vi "VI Main 1.1GPIB.vi"() -> ()   [LabVIEW 2014]
uses:
  <vilib>/Analysis/NI_AALPro.lvlib
panel:
  in  "clear graph at start":bool=TRUE
  in  "clear graph":bool
  out "Elapsed Time":dbl=5.100291728973389 format="%<%H:%M:%S>t"
  out "Measuring!":bool
  out "Current Interval":i32=2
  out "Benchmark (s)":dbl=1.077 format="%.2g"
  out "Start time":timestamp=timestamp(3634319869.0891385 s since 1904-01-01)
  in  "STOP acq":bool
  in  "# of Intervals":i32=20 min=2 step=1
  in  "Interval (s)":dbl=3.0 min=1.0 step=1.0
  in  "Quick Acq":bool
  in  "Multi Acq":bool
  in  "Reset":bool
  in  "Single Acq":bool
  in  "stop":bool
  out "intercept":dbl=5.632151768673284e-07 format="%_4g"
  out "Waveform Chart":dbl(graph)=1498.8953969009954
  out "Res. (ohm)":dbl=1498.8953969009954 format="%#.5g"
  out "XY Graph":cluster{dbl[], "Best Linear Fit":dbl[]}[](graph)=[{[0.0, 0.05050000175833702, 0.10100000351667404, 0.15150000154972076, 0.20200000703334808, 0.2524999976158142, 0.30300000309944153, 0.35350000858306885, 0.40400001406669617, 0.4544999897480011, 0.5049999952316284, 0.5554999709129333, 0.6060000061988831, 0.656499981880188, 0.7070000171661377, 0.7574999928474426, 0.8080000281333923, 0.8585000038146973, 0.9089999794960022, 0.9595000147819519, 1.0099999904632568, 1.0605000257492065, 1.1109999418258667, 1.1614999771118164, 1.2120000123977661, 1.2625000476837158, 1.312999963760376, 1.3634999990463257, 1.4140000343322754, 1.4644999504089355, 1.5149999856948853, 1.565500020980835, 1.6160000562667847, 1.6664999723434448, 1.7170000076293945, 1.7675000429153442, 1.8179999589920044, 1.868499994277954, 1.9190000295639038, 1.969499945640564, 2.0199999809265137, 2.070499897003174, 2.121000051498413, 2.1714999675750732, 2.2219998836517334, 2.2725000381469727, 2.322999954223633, 2.373500108718872, 2.4240000247955322, 2.4744999408721924, 2.5255000591278076, 2.5759999752044678, 2.626499891281128, 2.677000045776367, 2.7274999618530273, 2.7780001163482666, 2.8285000324249268, 2.878999948501587, 2.929500102996826, 2.9800000190734863, 3.0304999351501465, 3.0810000896453857, 3.131500005722046, 3.181999921798706, 3.2325000762939453, 3.2829999923706055, 3.3334999084472656, 3.384000062942505, 3.434499979019165, 3.484999895095825, 3.5355000495910645, 3.5859999656677246, 3.6364998817443848, 3.687000036239624, 3.737499952316284, 3.7880001068115234, 3.8385000228881836, 3.8889999389648438, 3.939500093460083, 3.990000009536743, 4.040500164031982, 4.091000080108643, 4.141499996185303, 4.191999912261963, 4.242499828338623, 4.293000221252441, 4.343500137329102, 4.394000053405762, 4.444499969482422, 4.494999885559082, 4.545499801635742, 4.5960001945495605, 4.646500110626221, 4.697000026702881, 4.747499942779541, 4.797999858856201, 4.848499774932861, 4.89900016784668, 4.94950008392334, 5.0], "Best Linear Fit"=[2.9321361694201187e-07, 3.4316144592594355e-05, 6.788442260585725e-05, 0.00010163152910536155, 0.0001353666593786329, 0.0001692490477580577, 0.00020289691747166216, 0.0002365230757277459, 0.0002702110796235502, 0.0003039317671209574, 0.0003375497763045132, 0.00037135041202418506, 0.00040501810144633055, 0.000438651826698333, 0.0004723611054942012, 0.0005059913382865489, 0.0005397166823968291, 0.0005734616424888372, 0.0006071235402487218, 0.0006408520275726914, 0.000674474285915494, 0.0007079437491483986, 0.0007418016903102398, 0.0007753406534902751, 0.0008092316566035151, 0.0008428616565652192, 0.0008766247192397714, 0.0009101884788833559, 0.0009441068395972252, 0.000977773917838931, 0.0010113242315128446, 0.00104525254573673, 0.0010786742204800248, 0.0011119291884824634, 0.0011458882363513112, 0.0011792887235060334, 0.0012128128437325358, 0.001246674102731049, 0.0012809749459847808, 0.0013138956855982542, 0.0013484194641932845, 0.0013821402098983526, 0.001415521022863686, 0.0014488088199868798, 0.0014823464443907142, 0.0015171199338510633, 0.0015507071511819959, 0.0015843959990888834, 0.0016174258198589087, 0.001652282546274364, 0.001685628667473793, 0.001718429964967072, 0.0017526380252093077, 0.0017857326893135905, 0.0018194534350186586, 0.001854273141361773, 0.0018880483694374561, 0.0019207267323508859, 0.0019549881108105183, 0.001989204902201891, 0.0020224947948008776, 0.002056337194517255, 0.0020900650415569544, 0.0021233297884464264, 0.0021574627608060837, 0.0021917179692536592, 0.0022237151861190796, 0.002258580643683672, 0.0022912463173270226, 0.0023252873215824366, 0.0023596647661179304, 0.0023923530243337154, 0.0024269770365208387, 0.0024603772908449173, 0.002494191052392125, 0.0025280059780925512, 0.0025607654824852943, 0.0025952423457056284, 0.0026286595966666937, 0.0026625576429069042, 0.002696041017770767, 0.002730145351961255, 0.0027635691221803427, 0.0027978394646197557, 0.00283193145878613, 0.0028640953823924065, 0.002898684237152338, 0.0029313690029084682, 0.002965638181194663, 0.0029995907098054886, 0.0030326275154948235, 0.0030669174157083035, 0.003100987756624818, 0.003135110717266798, 0.0031680287793278694, 0.0032008818816393614, 0.0032355813309550285, 0.003269442357122898, 0.0033022440038621426, 0.0033363213296979666]}, {[0.0, 0.05050000175833702, 0.10100000351667404, 0.15150000154972076, 0.20200000703334808, 0.2524999976158142, 0.30300000309944153, 0.35350000858306885, 0.40400001406669617, 0.4544999897480011, 0.5049999952316284, 0.5554999709129333, 0.6060000061988831, 0.656499981880188, 0.7070000171661377, 0.7574999928474426, 0.8080000281333923, 0.8585000038146973, 0.9089999794960022, 0.9595000147819519, 1.0099999904632568, 1.0605000257492065, 1.1109999418258667, 1.1614999771118164, 1.2120000123977661, 1.2625000476837158, 1.312999963760376, 1.3634999990463257, 1.4140000343322754, 1.4644999504089355, 1.5149999856948853, 1.565500020980835, 1.6160000562667847, 1.6664999723434448, 1.7170000076293945, 1.7675000429153442, 1.8179999589920044, 1.868499994277954, 1.9190000295639038, 1.969499945640564, 2.0199999809265137, 2.070499897003174, 2.121000051498413, 2.1714999675750732, 2.2219998836517334, 2.2725000381469727, 2.322999954223633, 2.373500108718872, 2.4240000247955322, 2.4744999408721924, 2.5255000591278076, 2.5759999752044678, 2.626499891281128, 2.677000045776367, 2.7274999618530273, 2.7780001163482666, 2.8285000324249268, 2.878999948501587, 2.929500102996826, 2.9800000190734863, 3.0304999351501465, 3.0810000896453857, 3.131500005722046, 3.181999921798706, 3.2325000762939453, 3.2829999923706055, 3.3334999084472656, 3.384000062942505, 3.434499979019165, 3.484999895095825, 3.5355000495910645, 3.5859999656677246, 3.6364998817443848, 3.687000036239624, 3.737499952316284, 3.7880001068115234, 3.8385000228881836, 3.8889999389648438, 3.939500093460083, 3.990000009536743, 4.040500164031982, 4.091000080108643, 4.141499996185303, 4.191999912261963, 4.242499828338623, 4.293000221252441, 4.343500137329102, 4.394000053405762, 4.444499969482422, 4.494999885559082, 4.545499801635742, 4.5960001945495605, 4.646500110626221, 4.697000026702881, 4.747499942779541, 4.797999858856201, 4.848499774932861, 4.89900016784668, 4.94950008392334, 5.0], "Best Linear Fit"=[5.632151768673284e-07, 3.425469348999516e-05, 6.794617180312299e-05, 0.00010163764763089373, 0.00013532912842937865, 0.0001690205992864352, 0.00020271208008492013, 0.00023640356088340506, 0.00027009504168188996, 0.0003037865025975182, 0.0003374779833960031, 0.00037116944431163135, 0.0004048609449929729, 0.00043855240590860115, 0.0004722439065899428, 0.000505935367505571, 0.0005396268681869126, 0.0005733183291025409, 0.0006070097900181691, 0.0006407012906995107, 0.0006743927516151388, 0.0007080842522964805, 0.0007417756734463953, 0.0007754671741277369, 0.0008091586748090786, 0.0008428501754904202, 0.000876541596640335, 0.0009102330973216766, 0.0009439245980030183, 0.000977616019152933, 0.0010113075198342747, 0.0010449990205156163, 0.001078690521196958, 0.0011123819423468728, 0.0011460734430282144, 0.001179764943709556, 0.0012134563648594707, 0.0012471478655408123, 0.001280839366222154, 0.0013145307873720688, 0.0013482222880534104, 0.0013819137092033252, 0.0014156052894160936, 0.0014492967105660085, 0.0014829881317159233, 0.0015166797119286917, 0.0015503711330786066, 0.001584062713291375, 0.0016177541344412898, 0.0016514455555912046, 0.0016854706906080038, 0.0017191621117579187, 0.0017528535329078335, 0.001786545113120602, 0.0018202365342705167, 0.0018539281144832852, 0.0018876195356332, 0.0019213109567831148, 0.001955002536995883, 0.001988693958145798, 0.0020223853792957127, 0.0020560769595084813, 0.002089768380658396, 0.002123459801808311, 0.002157151382021079, 0.0021908428031709943, 0.002224534224320909, 0.0022582258045336775, 0.002291917225683592, 0.002325608646833507, 0.0023593002270462754, 0.00239299164819619, 0.002426683069346105, 0.0024603746495588733, 0.0024940660707087883, 0.0025277576509215565, 0.0025614490720714716, 0.002595140493221386, 0.002628832073434155, 0.0026625234945840694, 0.002696215074796838, 0.0027299064959467527, 0.0027635979170966677, 0.0027972893382465823, 0.0028309807593964974, 0.002864672498672119, 0.0028983639198220342, 0.002932055340971949, 0.002965746762121864, 0.0029994381832717785, 0.0030331296044216935, 0.0030668213436973154, 0.0031005127648472304, 0.003134204185997145, 0.0031678956071470596, 0.0032015870282969747, 0.0032352784494468893, 0.0032689701887225115, 0.003302661609872426, 0.003336353031022341]}]
  in  "Sense range":i32(slide)
  in  "Stop (V)":dbl=5.0 format="%.4f"
  in  "Source compliance (A)":dbl=0.01 format="%.4f"
  in  "Direction":i32(slide)
  in  "Ranging":i32(slide)
  in  "Start (V)":dbl step=1.0 format="%.4p"
  in  "# of points to acquire":i32=50 min=1 max=2500 step=1
  in  "Speed":i32(slide)=2
  out "status":i32 format="%.0x"
  in  "resource name 2":string="GPIB0::24::INSTR"
  in  "resource name":string="ASRL4::INSTR"
  out "Qrun":bool
  out "Mrun":bool
  out "Srun":bool
  # ">"
  # "by L.Andrzejewski\nlandrzej@uottawa.ca"
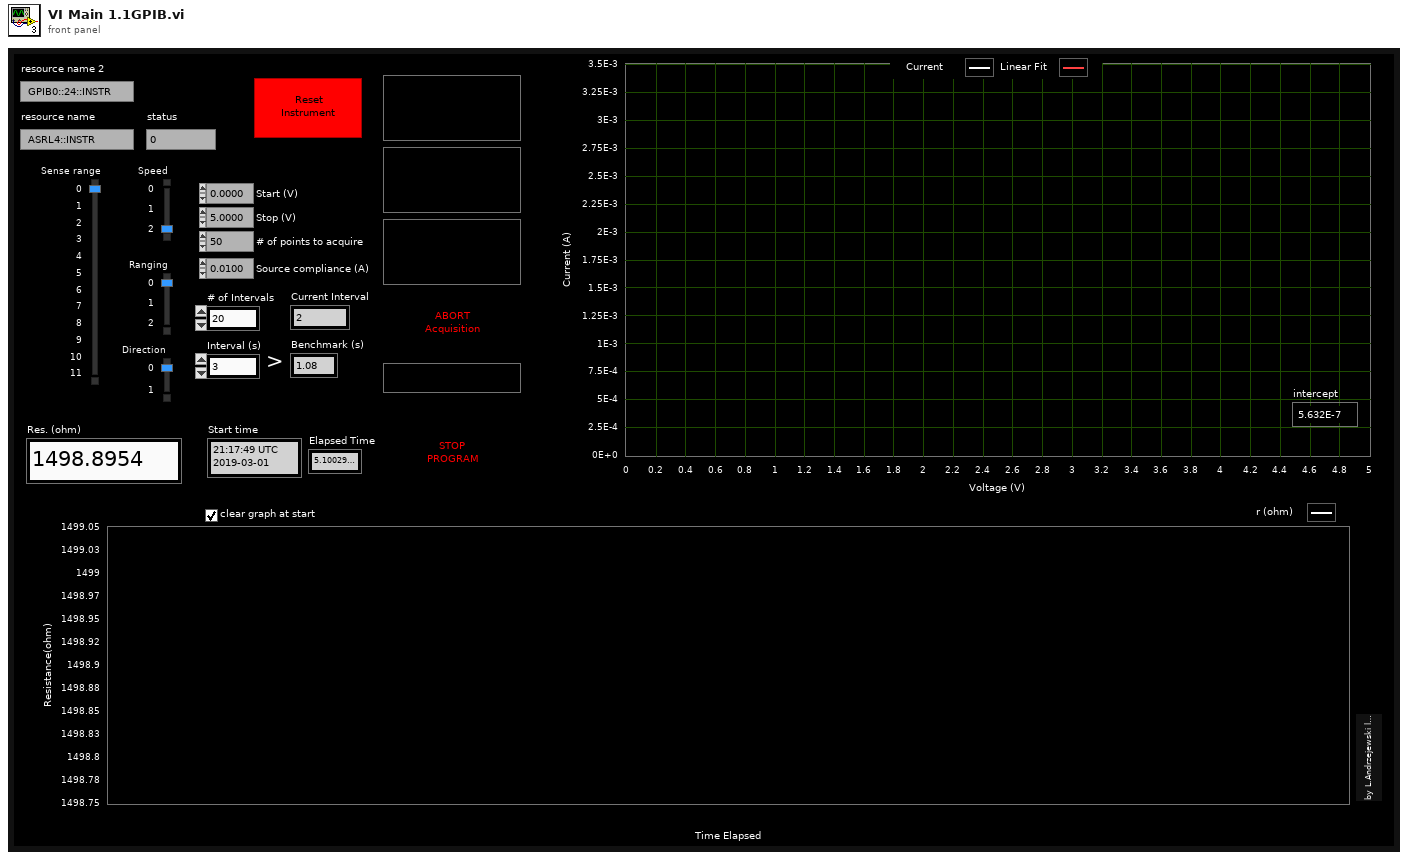
[diagram p1: front panel]
types:
  T1 = enum8{"Enabled", "Disabled", "Disabled and Grayed Out"}
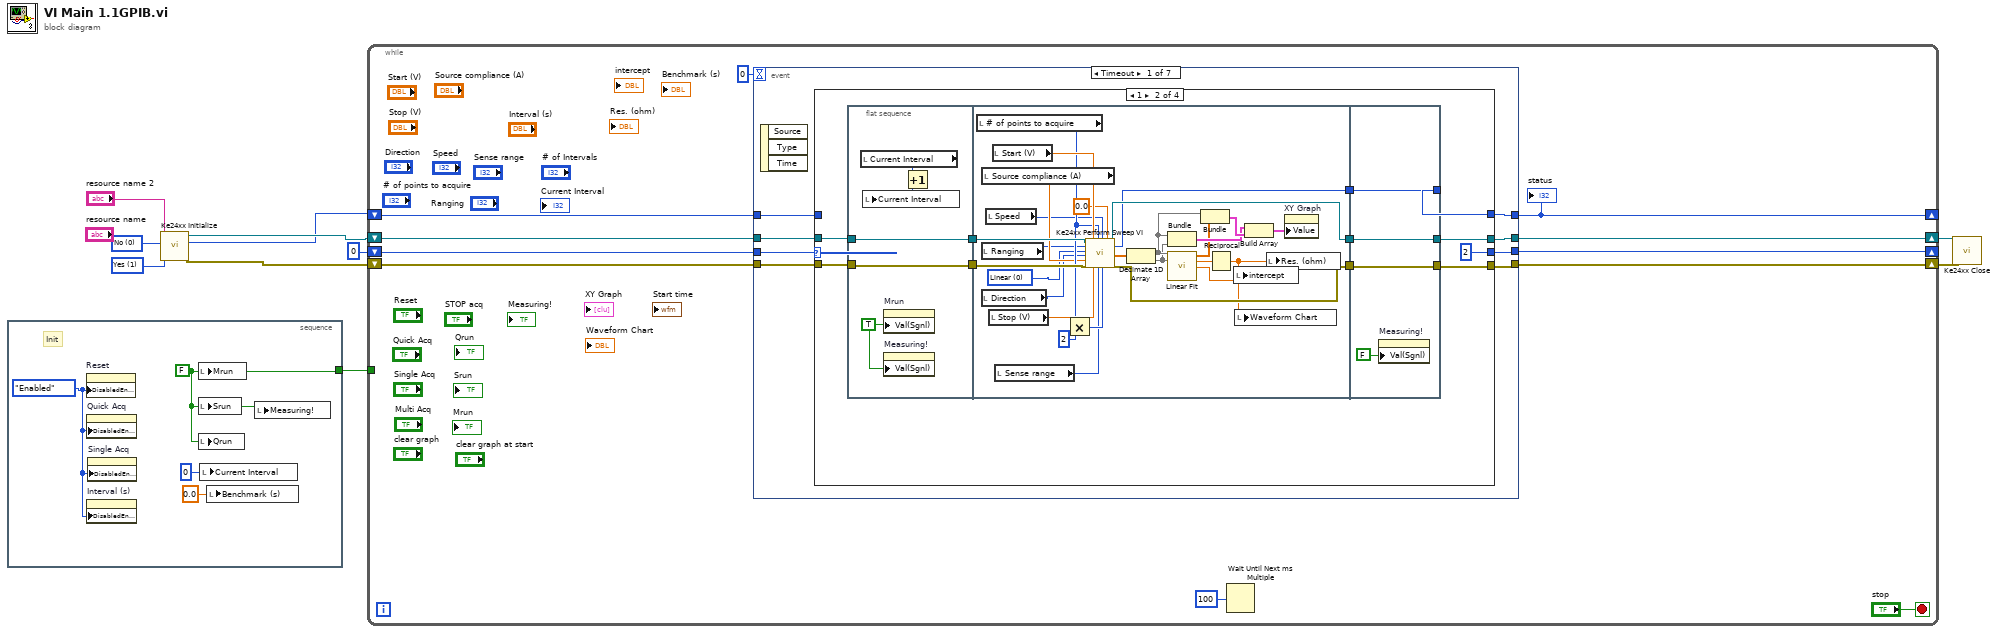
[diagram p0: block diagram]
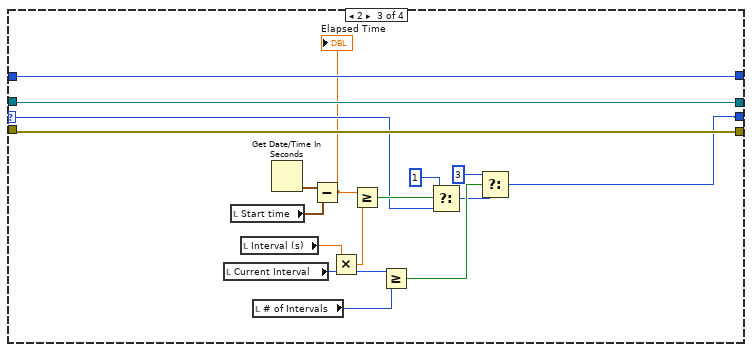
[diagram p3: hidden frame]
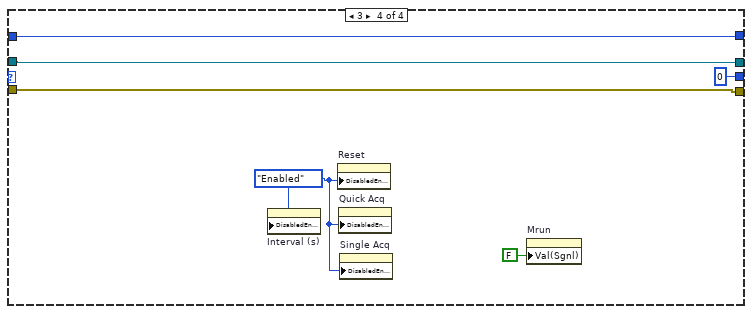
[diagram p4: hidden frame]
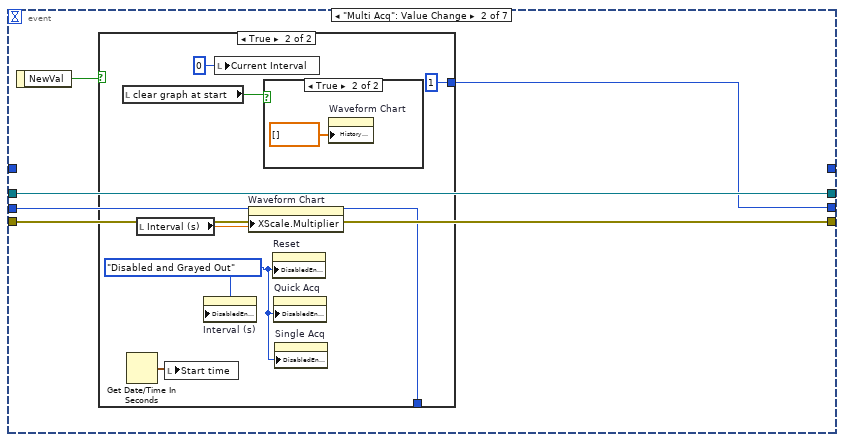
[diagram p5: hidden frame]
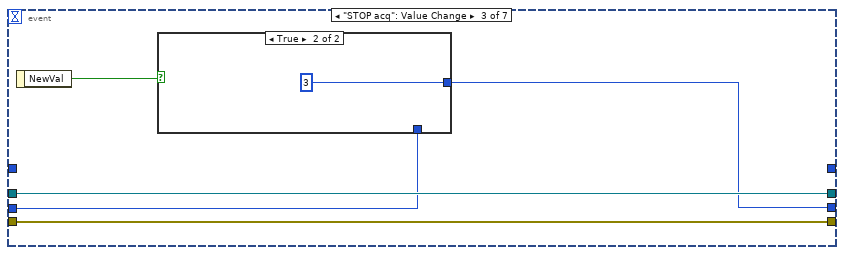
[diagram p8: hidden frame]
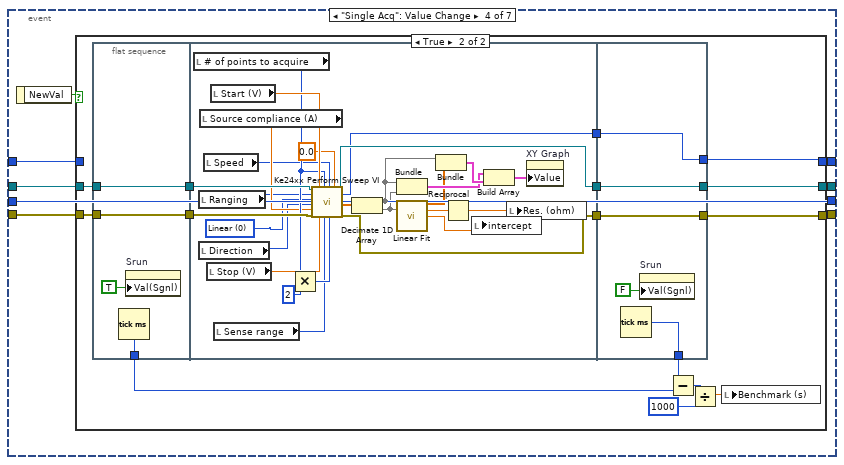
[diagram p10: hidden frame]
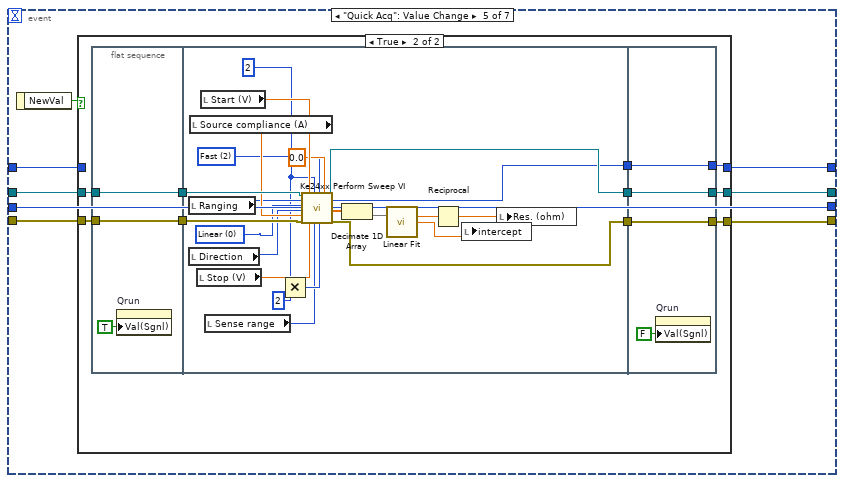
[diagram p12: hidden frame]
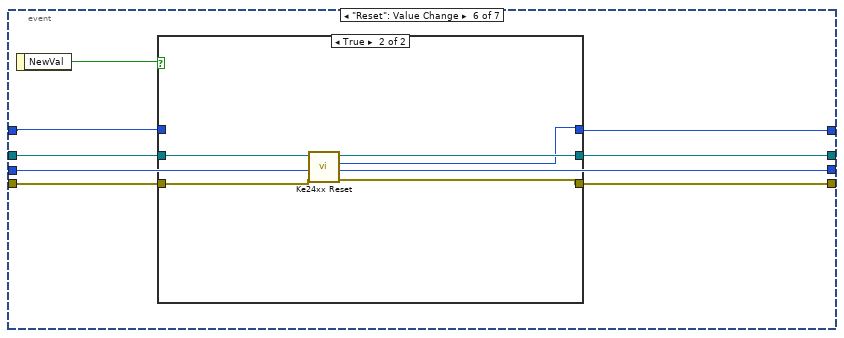
[diagram p14: hidden frame]
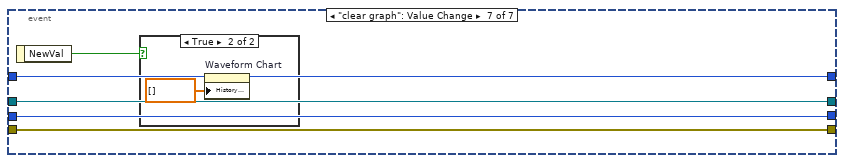
[diagram p16: hidden frame]
diagram:
  w9 = u16 1 items=["Yes"=1, "No"=0] ("id query")
  w10 = u16 0 items=["Yes"=1, "No"=0] ("reset device")
  n1 = stacked-sequence {
    tunnel: [w12] -> w3
    frame #0 {
      w11 = T1."Enabled" ("Disabled")
      w12 = FALSE ("Mrun")
      # "Init"
      n2 = property on="Reset" class="Bool"("DisabledEnum"=w11) -> ()  [unwired: 2 in, 2 out]
      n3 = property on="Quick Acq" class="Bool"("DisabledEnum"=w11) -> ()  [unwired: 2 in, 2 out]
      n4 = property on="Interval (s)" class="DigNum (strict)"("DisabledEnum"=w11) -> ()  [unwired: 2 in, 2 out]
      n5 = property on="Single Acq" class="Bool"("DisabledEnum"=w11) -> ()  [unwired: 2 in, 2 out]
      n6 = local write "Mrun"(w12) -> ()
      n7 = local write "Srun"(w12) -> ()
      n8 = local write "Qrun"(w12) -> ()
      n9 = local write "Current Interval"(0 ("Current Interval")) -> ()
      n10 = local write "Benchmark (s)"(0.0 ("Benchmark (s)")) -> ()
      n11 = local write "Measuring!"(w12) -> ()
    }
  }
  n12 = call <instrlib>:"Ke24xx Initialize.vi"("reset device"=w10, "id query"=w9, "resource name"="resource name 2") -> ("error out"=w4:errorcluster, "status"=w5:i32, "instrument handle out"=w6:refnum<visa-resource-name>)  [unwired: 6 in]
  n13 = while {
    shift-right: [w20] -> w8
    shift-left: w6 -> [w22]
    shift-right: [w19] -> w7
    shift-left: w4 -> [w21]
    shift-right: [w17] -> _
    shift-left: w5 -> [w18]
    tunnel: w3 -> [_]
    shift-right: [w15] -> _
    shift-left: 0 -> [w16]
    stop <- "stop" stop-if-true
    n14 = event shown="[0] Timeout" {
      selector: _ -> [_ _ _ _ _ _ _]
      dyn-events: _ -> [_ _ _ _ _ _ _]
      timeout: 0 -> [_ _ _ _ _ _ _]
      tunnel: [w29 w111 w124 w131 w193 w244 w259] -> w20
      tunnel: w22 -> [w32 w111 w124 w134 w196 w245 w259]
      tunnel: [w28 w110 w123 w132 w194 w243 w257] -> w19
      tunnel: w21 -> [w31 w110 w123 w133 w195 w242 w257]
      tunnel: w18 -> [w30 _ _ w130 w192 w247 w260]
      tunnel: [w26 _ _ w129 w191 w246 w260] -> w17
      tunnel: w16 -> [w33 w108 w121 w128 w190 w241 w258]
      tunnel: [w27 w109 w122 w128 w190 w241 w258] -> w15
      event Timeout {
        n15 = event-data() -> ()  [unwired: 1 in, 3 out]
        n16 = case shown="1" w33 {
          selector: w33 -> [w34 _ w90 _]
          tunnel: w32 -> [w36 w46 w99 w105]
          tunnel: w31 -> [w35 w45 w100 w103]
          tunnel: w30 -> [w37 _ w101 w106]
          tunnel: [w36 w44 w99 w105] -> w29
          tunnel: [w35 w43 w100 w103] -> w28
          tunnel: [w34 2 w87 0 ("t")] -> w27
          tunnel: [w37 w41 w101 w106] -> w26
          frame 0, Default {
          }
          frame 1 {
            n17 = flat-sequence {
              tunnel: w45 -> [w52]
              tunnel: w46 -> [w53]
              tunnel: [w53] -> w48
              tunnel: [w52] -> w47
              tunnel: w48 -> [w73]
              tunnel: w47 -> [w72]
              tunnel: [w71] -> w40
              tunnel: [w70] -> w39
              tunnel: [w55] -> w38
              tunnel: [w82] -> w41
              tunnel: [w83] -> w44
              tunnel: [w84] -> w43
              tunnel: w40 -> [w84]
              tunnel: w39 -> [w83]
              tunnel: w38 -> [w82]
              frame #0 {
                w49 = TRUE ("Value (Signaling)")
                n18 = local read "Current Interval"() -> (w50:i32)
                n19 = property on="Mrun" class="Bool (strict)"("Val(Sgnl)"=w49) -> ()  [unwired: 2 in, 2 out]
                n20 = property on="Measuring!" class="Bool (strict)"("Val(Sgnl)"=w49) -> ()  [unwired: 2 in, 2 out]
                n21 = Increment(x=w50) -> (x+1=w51:i32)
                n22 = local write "Current Interval"(w51) -> ()
              }
              frame #1 {
                w57 = 0 items=["Linear", "Logarithmic"] ("spacing")
                n23 = local read "# of points to acquire"() -> (w64:i32)
                n24 = local read "Ranging"() -> (w59:i32)
                n25 = local read "Direction"() -> (w58:i32)
                n26 = local read "Source compliance (A)"() -> (w61:dbl)
                n27 = local read "Speed"() -> (w60:i32)
                n28 = local read "Stop (V)"() -> (w66:dbl)
                n29 = local read "Start (V)"() -> (w67:dbl)
                n30 = local read "Sense range"() -> (w62:i32)
                n31 = Multiply(x=w64, y=2) -> (x*y=w63:i32)
                n32 = call <instrlib>:"Ke24xx Perform Sweep VI.vi"("instrument handle"=w73, "ranging"=w59, "spacing"=w57, "direction"=w58, "source compliance"=w61, "error in (no error)"=w72, "start"=w67, "stop"=w66, "number of points"=w64, "sense range"=w62, "speed"=w60, "size of reading"=w63, "source protection"=0.0) -> ("instrument handle out"=w70:refnum<visa-resource-name>, "status"=w55:i32, "out"=w74:dbl[], "error out"=w71:errorcluster)  [unwired: 3 in]
                n33 = Decimate 1D Array(w74) -> (w78:dbl[], w75:dbl[])
                n34 = Bundle(w78, w75) -> (w79:cluster{dbl[], dbl[]})  [unwired: 1 in]
                n35 = call <vilib>:"Linear Fit.vi"("Y"=w75, "X"=w78) -> ("Best Linear Fit"=w77:dbl[], "slope"=w76:dbl, "intercept"=w69:dbl)  [unwired: 9 in, 2 out]
                n36 = Bundle(w78, "Best Linear Fit"=w77) -> (w80:cluster{dbl[], "Best Linear Fit":dbl[]})  [unwired: 1 in]
                n37 = Reciprocal(x=w76) -> (1/x=w54:dbl)
                n38 = local write "intercept"(w69) -> ()
                n39 = local write "Waveform Chart"(w54) -> ()
                n40 = Build Array(w79, w80) -> (w68:cluster{dbl[], "Best Linear Fit":dbl[]}[])
                n41 = local write "Res. (ohm)"(w54) -> ()
                n42 = property on="XY Graph" class="XYGraph (strict)"("Value"=w68) -> ()  [unwired: 2 in, 2 out]
              }
              frame #2 {
                n43 = property on="Measuring!" class="Bool (strict)"("Val(Sgnl)"=FALSE ("Value (Signaling)")) -> ()  [unwired: 2 in, 2 out]
              }
            }
          }
          frame 2 {
            n44 = local read "Current Interval"() -> (w93:i32)
            n45 = local read "Start time"() -> (w97:timestamp)
            n46 = local read "Interval (s)"() -> (w96:dbl)
            n47 = local read "# of Intervals"() -> (w92:i32)
            n48 = Get Date/Time In Seconds() -> (seconds since 1Jan1904=w98:timestamp)
            n49 = Subtract(x=w98, y=w97) -> (x-y=w85:dbl)
            "Elapsed Time" <- w85
            n50 = Multiply(x=w96, y=w93) -> (x*y=w95:dbl)
            n51 = Greater Or Equal?(x=w85, y=w95) -> (x >= y?=w94:bool)
            n52 = Greater Or Equal?(x=w93, y=w92) -> (x >= y?=w89:bool)
            n53 = Select(t=1, s=w94, f=w90) -> (s? t:f=w88:i32)
            n54 = Select(t=3, s=w89, f=w88) -> (s? t:f=w87:i32)
          }
          frame 3 {
            w102 = T1."Enabled" ("Disabled")
            n55 = property on="Interval (s)" class="DigNum (strict)"("DisabledEnum"=w102) -> ()  [unwired: 2 in, 2 out]
            n56 = property on="Reset" class="Bool"("DisabledEnum"=w102) -> ()  [unwired: 2 in, 2 out]
            n57 = property on="Quick Acq" class="Bool"("DisabledEnum"=w102) -> ()  [unwired: 2 in, 2 out]
            n58 = property on="Single Acq" class="Bool"("DisabledEnum"=w102) -> ()  [unwired: 2 in, 2 out]
            n59 = property on="Mrun" class="Bool (strict)"("Val(Sgnl)"=FALSE ("Value (Signaling)")) -> ()  [unwired: 2 in, 2 out]
          }
        }
      }
      event "Multi Acq": Value Change {
        n60 = event-data() -> ("NewVal"=w112:bool)  [unwired: 1 in]
        n61 = case shown="True" w112 {
          tunnel: [w113 1] -> w109
          tunnel: w108 -> [w113 _]
          frame False {
          }
          frame True {
            w115 = T1."Disabled and Grayed Out" ("Disabled")
            n62 = local read "clear graph at start"() -> (w114:bool)
            n63 = Get Date/Time In Seconds() -> (seconds since 1Jan1904=w117:timestamp)
            n64 = local read "Interval (s)"() -> (w116:dbl)
            n65 = local write "Start time"(w117) -> ()
            n66 = property on="Interval (s)" class="DigNum (strict)"("DisabledEnum"=w115) -> ()  [unwired: 2 in, 2 out]
            n67 = local write "Current Interval"(0 ("Current Interval")) -> ()
            n68 = property on="Waveform Chart" class="WFChart (strict)"("XScale.Multiplier"=w116) -> ()  [unwired: 2 in, 2 out]
            n69 = case shown="True" w114 {
              frame False {
              }
              frame True {
                n70 = property on="Waveform Chart" class="WFChart (strict)"("History Data"=dbl[] []) -> ()  [unwired: 2 in, 2 out]
              }
            }
            n71 = property on="Reset" class="Bool"("DisabledEnum"=w115) -> ()  [unwired: 2 in, 2 out]
            n72 = property on="Quick Acq" class="Bool"("DisabledEnum"=w115) -> ()  [unwired: 2 in, 2 out]
            n73 = property on="Single Acq" class="Bool"("DisabledEnum"=w115) -> ()  [unwired: 2 in, 2 out]
          }
        }
      }
      event "STOP acq": Value Change {
        n74 = event-data() -> ("NewVal"=w125:bool)  [unwired: 1 in]
        n75 = case shown="True" w125 {
          tunnel: [w126 3] -> w122
          tunnel: w121 -> [w126 _]
          frame False {
          }
          frame True {
          }
        }
      }
      event "Single Acq": Value Change {
        n76 = event-data() -> ("NewVal"=w135:bool)  [unwired: 1 in]
        n77 = case shown="True" w135 {
          tunnel: w134 -> [w138 w153]
          tunnel: w133 -> [w137 w152]
          tunnel: [w137 w151] -> w132
          tunnel: [w138 w150] -> w131
          tunnel: [w136 w145] -> w129
          tunnel: w130 -> [w136 _]
          frame False {
          }
          frame True {
            n78 = flat-sequence {
              tunnel: w152 -> [w156]
              tunnel: w153 -> [w157]
              tunnel: [w157] -> w147
              tunnel: [w156] -> w146
              tunnel: [w154] -> w142
              tunnel: [w175] -> w149
              tunnel: [w174] -> w148
              tunnel: w147 -> [w177]
              tunnel: w146 -> [w176]
              tunnel: [w158] -> w144
              tunnel: [w188] -> w150
              tunnel: [w189] -> w151
              tunnel: w149 -> [w189]
              tunnel: w148 -> [w188]
              tunnel: [w187] -> w145
              tunnel: w144 -> [w187]
              tunnel: [w185] -> w143
              frame #0 {
                n79 = Tick Count (ms)() -> (millisecond timer value=w154:u32)
                n80 = property on="Srun" class="Bool (strict)"("Val(Sgnl)"=TRUE ("Value (Signaling)")) -> ()  [unwired: 2 in, 2 out]
              }
              frame #1 {
                w160 = 0 items=["Linear", "Logarithmic"] ("spacing")
                n81 = local read "# of points to acquire"() -> (w167:i32)
                n82 = local read "Ranging"() -> (w162:i32)
                n83 = local read "Direction"() -> (w161:i32)
                n84 = local read "Source compliance (A)"() -> (w164:dbl)
                n85 = local read "Speed"() -> (w163:i32)
                n86 = local read "Stop (V)"() -> (w169:dbl)
                n87 = local read "Start (V)"() -> (w170:dbl)
                n88 = local read "Sense range"() -> (w165:i32)
                n89 = Multiply(x=w167, y=2) -> (x*y=w166:i32)
                n90 = call <instrlib>:"Ke24xx Perform Sweep VI.vi"("instrument handle"=w177, "ranging"=w162, "spacing"=w160, "direction"=w161, "source compliance"=w164, "error in (no error)"=w176, "start"=w170, "stop"=w169, "number of points"=w167, "sense range"=w165, "speed"=w163, "size of reading"=w166, "source protection"=0.0) -> ("instrument handle out"=w174:refnum<visa-resource-name>, "status"=w158:i32, "out"=w178:dbl[], "error out"=w175:errorcluster)  [unwired: 3 in]
                n91 = Decimate 1D Array(w178) -> (w182:dbl[], w179:dbl[])
                n92 = Bundle(w182, w179) -> (w183:cluster{dbl[], dbl[]})  [unwired: 1 in]
                n93 = call <vilib>:"Linear Fit.vi"("Y"=w179, "X"=w182) -> ("Best Linear Fit"=w181:dbl[], "slope"=w180:dbl, "intercept"=w173:dbl)  [unwired: 9 in, 2 out]
                n94 = Bundle(w182, "Best Linear Fit"=w181) -> (w184:cluster{dbl[], "Best Linear Fit":dbl[]})  [unwired: 1 in]
                n95 = Reciprocal(x=w180) -> (1/x=w172:dbl)
                n96 = local write "intercept"(w173) -> ()
                n97 = Build Array(w183, w184) -> (w171:cluster{dbl[], "Best Linear Fit":dbl[]}[])
                n98 = local write "Res. (ohm)"(w172) -> ()
                n99 = property on="XY Graph" class="XYGraph (strict)"("Value"=w171) -> ()  [unwired: 2 in, 2 out]
              }
              frame #2 {
                n100 = Tick Count (ms)() -> (millisecond timer value=w185:u32)
                n101 = property on="Srun" class="Bool (strict)"("Val(Sgnl)"=FALSE ("Value (Signaling)")) -> ()  [unwired: 2 in, 2 out]
              }
            }
            n102 = Subtract(x=w143, y=w142) -> (x-y=w141:u32)
            n103 = Divide(x=w141, y=u32 1000) -> (x/y=w139:dbl)
            n104 = local write "Benchmark (s)"(w139) -> ()
          }
        }
      }
      event "Quick Acq": Value Change {
        n105 = event-data() -> ("NewVal"=w197:bool)  [unwired: 1 in]
        n106 = case shown="True" w197 {
          tunnel: w196 -> [w200 w210]
          tunnel: w195 -> [w199 w209]
          tunnel: [w199 w208] -> w194
          tunnel: [w200 w207] -> w193
          tunnel: [w198 w202] -> w191
          tunnel: w192 -> [w198 _]
          frame False {
          }
          frame True {
            n107 = flat-sequence {
              tunnel: w209 -> [w212]
              tunnel: w210 -> [w213]
              tunnel: [w213] -> w206
              tunnel: [w212] -> w205
              tunnel: w206 -> [w232]
              tunnel: w205 -> [w231]
              tunnel: [w230] -> w204
              tunnel: [w229] -> w203
              tunnel: [w214] -> w201
              tunnel: [w239] -> w207
              tunnel: [w240] -> w208
              tunnel: w204 -> [w240]
              tunnel: w203 -> [w239]
              tunnel: [w237] -> w202
              tunnel: w201 -> [w237]
              frame #0 {
                n108 = property on="Qrun" class="Bool (strict)"("Val(Sgnl)"=TRUE ("Qrun")) -> ()  [unwired: 2 in, 2 out]
              }
              frame #1 {
                w215 = 2 items=["Slow", "Medium", "Fast"] ("speed")
                w216 = 2 ("x")
                w218 = 0 items=["Linear", "Logarithmic"] ("spacing")
                n109 = local read "Ranging"() -> (w220:i32)
                n110 = local read "Direction"() -> (w219:i32)
                n111 = local read "Source compliance (A)"() -> (w221:dbl)
                n112 = local read "Stop (V)"() -> (w225:dbl)
                n113 = local read "Start (V)"() -> (w226:dbl)
                n114 = local read "Sense range"() -> (w222:i32)
                n115 = Multiply(x=w216, y=2) -> (x*y=w223:i32)
                n116 = call <instrlib>:"Ke24xx Perform Sweep VI.vi"("instrument handle"=w232, "ranging"=w220, "spacing"=w218, "direction"=w219, "source compliance"=w221, "error in (no error)"=w231, "start"=w226, "stop"=w225, "number of points"=w216, "sense range"=w222, "speed"=w215, "size of reading"=w223, "source protection"=0.0) -> ("instrument handle out"=w229:refnum<visa-resource-name>, "status"=w214:i32, "out"=w233:dbl[], "error out"=w230:errorcluster)  [unwired: 3 in]
                n117 = Decimate 1D Array(w233) -> (w236:dbl[], w234:dbl[])
                n118 = call <vilib>:"Linear Fit.vi"("Y"=w234, "X"=w236) -> ("slope"=w235:dbl, "intercept"=w228:dbl)  [unwired: 9 in, 3 out]
                n119 = Reciprocal(x=w235) -> (1/x=w227:dbl)
                n120 = local write "intercept"(w228) -> ()
                n121 = local write "Res. (ohm)"(w227) -> ()
              }
              frame #2 {
                n122 = property on="Qrun" class="Bool (strict)"("Val(Sgnl)"=FALSE ("Qrun")) -> ()  [unwired: 2 in, 2 out]
              }
            }
          }
        }
      }
      event "Reset": Value Change {
        n123 = event-data() -> ("NewVal"=w248:bool)  [unwired: 1 in]
        n124 = case shown="True" w248 {
          tunnel: [w251 w252] -> w246
          tunnel: w247 -> [w251 _]
          tunnel: w245 -> [w250 w256]
          tunnel: [w250 w255] -> w244
          tunnel: [w249 w253] -> w243
          tunnel: w242 -> [w249 w254]
          frame False {
          }
          frame True {
            n125 = call <instrlib>:"Ke24xx Reset.vi"("error in (no error)"=w254, "instrument handle"=w256) -> ("error out"=w253:errorcluster, "status"=w252:i32, "instrument handle out"=w255:refnum<visa-resource-name>)  [unwired: 7 in]
          }
        }
      }
      event "clear graph": Value Change {
        n126 = event-data() -> ("NewVal"=w261:bool)  [unwired: 1 in]
        n127 = case shown="True" w261 {
          frame False {
          }
          frame True {
            n128 = property on="Waveform Chart" class="WFChart (strict)"("History Data"=dbl[] []) -> ()  [unwired: 2 in, 2 out]
          }
        }
      }
    }
    "status" <- w17
    n129 = Wait Until Next ms Multiple(millisecond multiple=u32 100) -> ()  [unwired: 1 out]
  }
  n130 = call <instrlib>:"Ke24xx Close.vi"("error in (no error)"=w7, "instrument handle"=w8) -> ()  [unwired: 8 in, 2 out]
